vi "PS_ENABLE_OUTPUT.vi"(4 "CH4":bool, 6 "CH3":bool, 8 "error in (no error)":errorcluster {"code" format="%.0x"}, 11 "VISA resource name":refnum<visa-resource-name>) -> (0 "error out":errorcluster {"code" format="%.0x"})   [LabVIEW 2018]
uses:
  Agilent N6700 Series/Agilent N6700 Series.lvlib
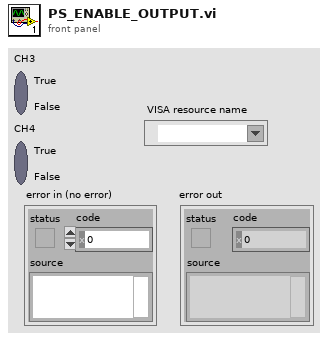
[diagram p1: front panel]
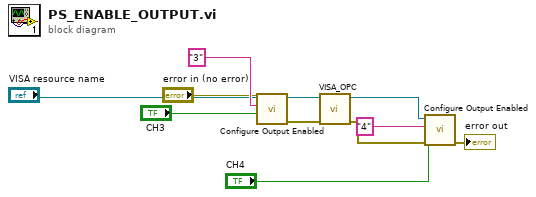
[diagram p0: block diagram]
diagram:
  n1 = call "Configure Output Enabled.vi"("error in (no error)"="error in (no error)", "Enable Output (False)"="CH3", "Channel Name (1)"="3", "VISA resource name"="VISA resource name") -> ("error out"=w8:errorcluster, "VISA resource name out"=w3:refnum<visa-resource-name>)  [unwired: 6 in]
  n2 = call "VISA_OPC.vi"("error in"=w8, "Session In"=w3) -> ("error out"=w9:errorcluster, "Session Out"=w11:refnum<visa-resource-name>)  [unwired: 7 in, 1 out]
  n3 = call "Configure Output Enabled.vi"("error in (no error)"=w9, "Enable Output (False)"="CH4", "Channel Name (1)"="4", "VISA resource name"=w11) -> ("error out"=→"error out":errorcluster)  [unwired: 6 in, 1 out]
